vi "Add VI or CTL to lvlib or lvclass.vi"(8 "error in":errorcluster, 10 "VI Ref":refnum<vi>, 11 "lvlib or lvclass Ref":refnum<vi>) -> (0 "error out":errorcluster)   [LabVIEW 2022 SP3]
doc: "<add doc>"
panel:
  # "Development\ncontrols/indicators useful for development and testing, but which are not outputs of the VI"
  # "Input\nInputs to the VI"
  # "Output\nOutputs of the VI"
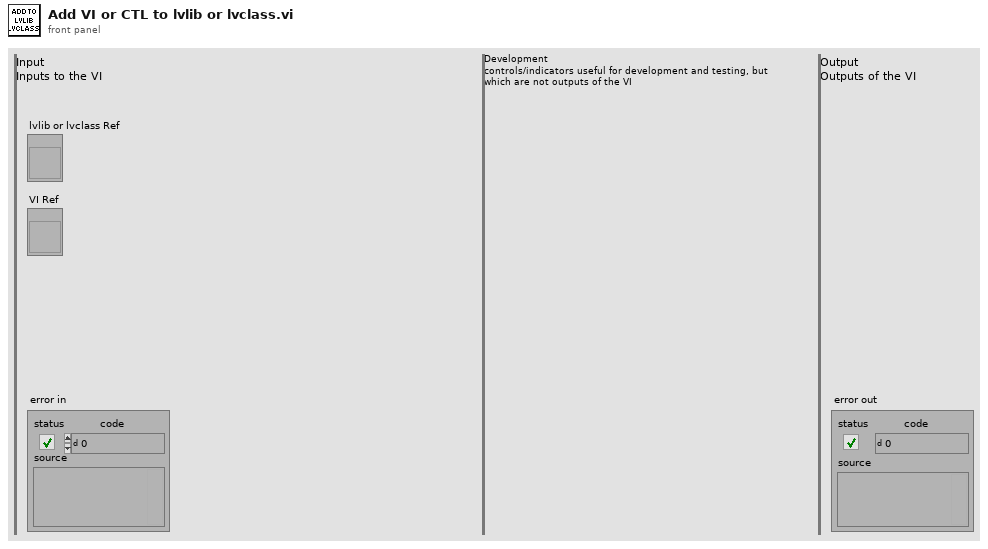
[diagram p1: front panel]
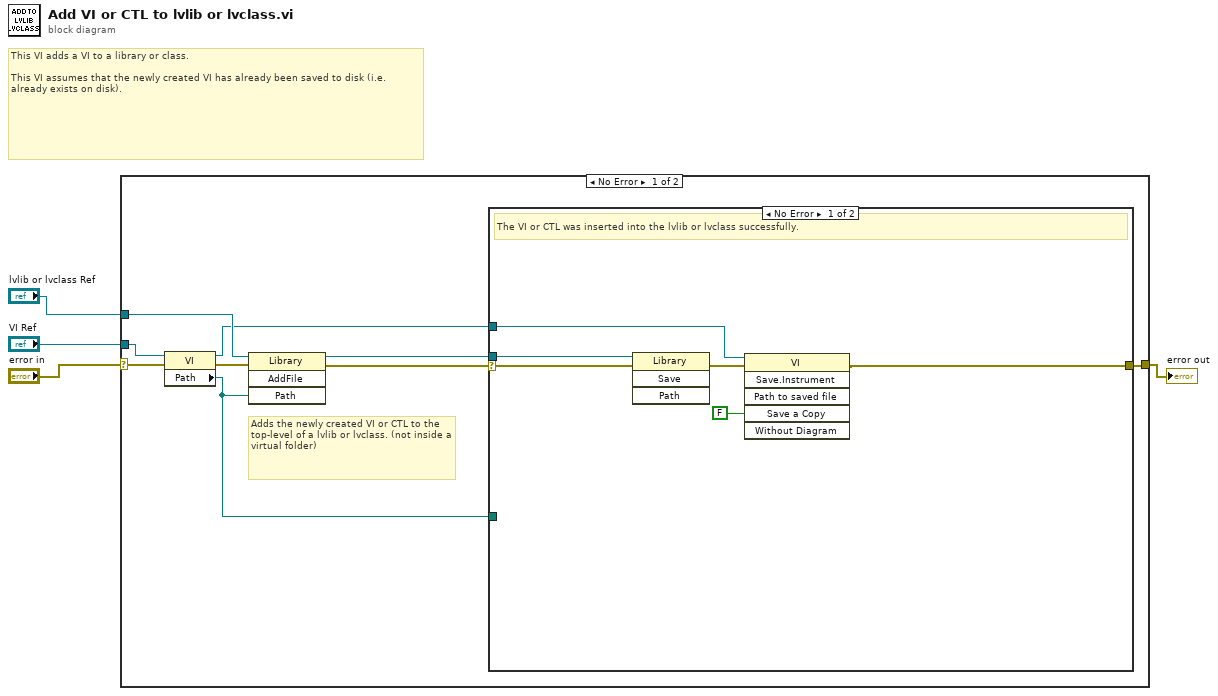
[diagram p0: block diagram]
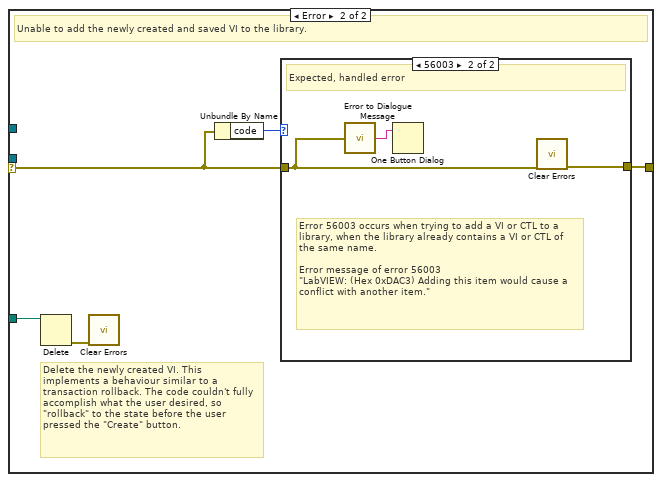
[diagram p2: hidden frame]
diagram:
  # "This VI adds a VI to a library or class.\n\nThis VI assumes that the newly created VI has already been saved to disk (i.e. already exists on disk)."
  n1 = case shown="No Error" "error in" {
    selector: "error in" -> [w13 w29]
    tunnel: [w12 w29] -> w3
    tunnel: "lvlib or lvclass Ref" -> [w7 _]
    tunnel: "VI Ref" -> [w5 _]
    frame No Error {
      # "Adds the newly created VI or CTL to the top-level of a lvlib or lvclass. (not inside a virtual folder)"
      n2 = property class="VI"(reference=w5, error in=w13) -> (reference out=w6:refnum<vi>, error out=w10:errorcluster, "Path"=w9:path)
      n3 = invoke class="Library" method="AddFile"(reference=w7, error in=w10, "Path"=w9) -> (reference out=w8:refnum<vi>, error out=w11:errorcluster)  [unwired: 1 in, 2 out]
      n4 = case shown="No Error" w11 {
        selector: w11 -> [w19 w22]
        tunnel: w8 -> [w17 _]
        tunnel: [w16 w23] -> w12
        tunnel: w6 -> [w15 _]
        tunnel: w9 -> [_ w21]
        frame No Error {
          # "The VI or CTL was inserted into the lvlib or lvclass successfully."
          n5 = invoke class="Library" method="Save"(reference=w17, error in=w19) -> (error out=w18:errorcluster)  [unwired: 2 in, 3 out]
          n6 = invoke class="VI" method="Save.Instrument"(reference=w15, error in=w18, "Save a Copy"=FALSE) -> (error out=w16:errorcluster)  [unwired: 3 in, 5 out]
        }
        frame Error {
          # "Delete the newly created VI. This implements a behaviour similar to a transaction rollback. The code couldn't fully accomplish what the user desired, so \"rollback\" to the state before the user pressed the \"Create\" button."
          # "Unable to add the newly created and saved VI to the library."
          n7 = Delete(path (use dialog)=w21) -> (error out=w20:errorcluster)  [unwired: 4 in, 2 out]
          n8 = call <vilib>:"Clear Errors.vi"("error in (no error)"=w20) -> ()  [unwired: 5 in, 2 out]
          n9 = Unbundle By Name(w22) -> ("code"=w24:i32)
          n10 = case shown="56003" w24 {
            tunnel: w22 -> [w25 w27]
            tunnel: [w25 w28] -> w23
            frame Default {
              # "Do nothing. The error will be handled downstream."
              # "Unexpected error"
            }
            frame 56003 {
              # "Error 56003 occurs when trying to add a VI or CTL to a library, when the library already contains a VI or CTL of the same name.\n\nError message of error 56003\n\"LabVIEW: (Hex 0xDAC3) Adding this item would cause a conflict with another item.\""
              # "Expected, handled error"
              n11 = call "Error to Dialogue Message.vi"("error in"=w27) -> ("Dialogue Message"=w26:string)
              n12 = One Button Dialog(message=w26) -> ()  [unwired: 1 in, 1 out]
              n13 = call <vilib>:"Clear Errors.vi"("error in (no error)"=w27) -> ("error out"=w28:errorcluster)  [unwired: 5 in, 1 out]
            }
          }
        }
      }
    }
    frame Error {
    }
  }
  "error out" <- w3
